vi "Is IPv4 Address IPv4LL.vi"(11 "address":refnum<class "IPv4 Network Address.lvclass">) -> (3 "IPv4LL?":bool)   [LabVIEW 2020, in "NI_WFCN.lvlib" / "IPv4 Network Address.lvclass"]
doc: "Does this address fall in the IPv4LL range (169.254.0.0/16)? Address is in native-byte-order U32 format."
uses:
  <vilib>/net/WFCN/Addressing/IPv4 Network Address/IPv4 Network Address.lvclass
  <vilib>/net/WFCN/Addressing/IPv4 Network Address/IPv4 Network Address.lvclass/IPv4 Network Address.ctl
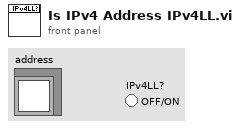
[diagram p1: front panel]
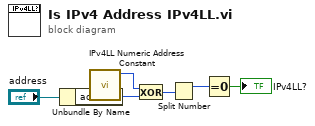
[diagram p0: block diagram]
diagram:
  n1 = Unbundle By Name("address") -> ("address"=w1:u32)
  n2 = call <vilib>:"IPv4LL Numeric Address Constant.vi"() -> ("IPv4LL Subnet Address"=w6:u32)  [unwired: 11 in]
  n3 = Exclusive Or(1:w1, 2:w6) -> (0:w5:u32)
  n4 = Split Number(x=w5) -> (hi(x)=w4:u16)  [unwired: 1 out]
  n5 = Equal To 0?(x=w4) -> (x = 0?=→"IPv4LL?":bool)
